vi "ConfigureAppender.vi"(5 "filter":T1={"mode"=enum."Mirror", "levelMin"=enum."INFO", "levelMax"=enum."INFO", "tagPrefix"=""}, 7 "threshold":T3=enum."INFO", 8 "error in (no error)":errorcluster, 10 "id":string, 11 "LogManager in":refnum<class "LogManager.lvclass">) -> (0 "error out":errorcluster, 3 "LogManager out":refnum<class "LogManager.lvclass">)   [LabVIEW 2026, in "Lumberjack.lvlib" / "LogManager.lvclass"]
doc: "Forward a gate reconfiguration (threshold + filter) to a specific appender identified by id. Looks the appender up in the registry (FindByID); if found, sends a ConfigureMsg to its enqueuer so the appender updates its own gate; if not found, warns gracefully (status FALSE) and does nothing. Does not mutate manager state and does not post the Snapshot (per-appender gate is not in the Snapshot). Called by ConfigureAppenderMsg:Do (SRS-LMBR-047)."
uses:
  LogManager.lvclass
  TypeDefs/Severity.ctl
  TypeDefs/Filter.ctl
  TypeDefs/FilterMode.ctl
  LogManager.lvclass/LogManager.ctl
  Messages/ConfigureMsg.lvclass/ConfigureMsg.lvclass
  Lumberjack.lvlib
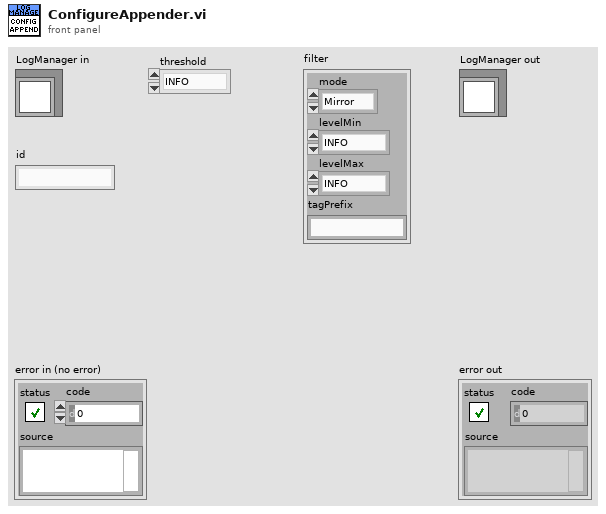
[diagram p1: front panel]
types:
  T1 = typedef "Lumberjack.lvlib/Filter.ctl" = cluster{"mode":T2, "levelMin":T3, "levelMax":T3, "tagPrefix":string}
  T2 = typedef "Lumberjack.lvlib/FilterMode.ctl" = enum16{"Mirror", "Routed"}
  T3 = typedef "Lumberjack.lvlib/Severity.ctl" = enum16{"OFF", "FATAL", "ERROR", "WARN", "INFO", "DEBUG", "TRACE", "ALL"}
  T4 = typedef "Lumberjack.lvlib/RegistryEntry.ctl" = cluster{"id":string, "enqueuer":refnum<class "Message Enqueuer.lvclass">}
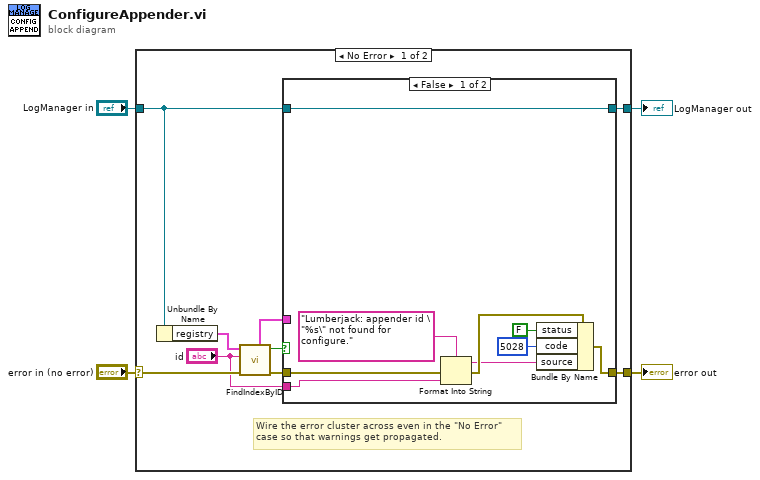
[diagram p0: block diagram]
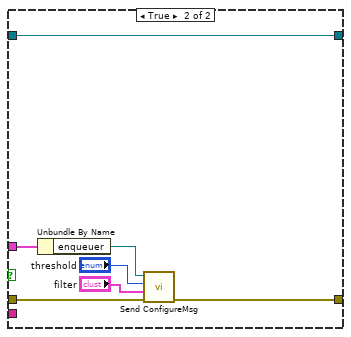
[diagram p2: hidden frame]
diagram:
  n1 = case shown="No Error" "error in (no error)" {
    selector: "error in (no error)" -> [w12 w31]
    tunnel: [w8 w31] -> w3
    tunnel: [w9 w30] -> w1
    tunnel: "LogManager in" -> [w11 w30]
    frame No Error {
      # "Wire the error cluster across even in the \"No Error\"\ncase so that warnings get propagated."
      n2 = Unbundle By Name(w11) -> ("registry"=w13:T4[])
      n3 = call "FindIndexByID.vi"("error in (no error)"=w12, "id"="id", "registry"=w13) -> ("error out"=w10:errorcluster, "found"=w7:bool, "registryEntry"=w6:T4)  [unwired: 5 in, 1 out]
      n4 = case shown="False" w7 {
        tunnel: w11 -> [w22 w29]
        tunnel: w10 -> [w16 w26]
        tunnel: [w22 w29] -> w9
        tunnel: [w15 w27] -> w8
        tunnel: w6 -> [_ w28]
        tunnel: "id" -> [w14 _]
        frame False {
          n5 = Format Into String(format string="Lumberjack: appender id \"%s\" not found for configure." ("source"), error in=w16, w14) -> (resulting string=w20:string, error out=w21:errorcluster)  [unwired: 1 in]
          n6 = Bundle By Name(cluster=w21, "status"=FALSE, "code"=5028, "source"=w20) -> (w15:errorcluster)
        }
        frame True {
          n7 = Unbundle By Name(w28) -> ("enqueuer"=w25:refnum<class "Message Enqueuer.lvclass">)
          n8 = call "Send ConfigureMsg.vi"("error in (no error)"=w26, "filter"="filter", "threshold"="threshold", "Enqueuer in"=w25) -> ("error out"=w27:errorcluster)  [unwired: 6 in, 1 out]
        }
      }
    }
    frame Error {
    }
  }
  "error out" <- w3
  "LogManager out" <- w1
